vi "Pose3d_getRotation3d.vi"(11 "in Pose3d":T3={"Translation3d"={"X"=0.0, "Y"=0.0, "Z"=0.0}, "Rotation3d"={"Q_quaternion"={"R"=1.0, "V"=[0.0, 0.0, 0.0]}}} {"Translation3d"."Z" format="%14.3f"; "Translation3d"."Y" format="%14.3f"; "Translation3d"."X" format="%14.3f"}) -> (3 "out Rotation3d":T1={"Q_quaternion"={"R"=1.0, "V"=[0.0, 0.0, 0.0]}})   [LabVIEW 2019, in "Trajectory_Library.lvlib"]
doc: "Returns the rotational component of the transformation.\n\nParmeters:\n - IN POSE -- Input POSE data structure\n\nRETURNS:\n - out ROTATION - The rotational component of the pose."
uses:
  Trajectory_Library.lvlib
  POSE3D.ctl
  TRANSLATION3D.ctl
  ROTATION3D.ctl
  QUATERNION.ctl
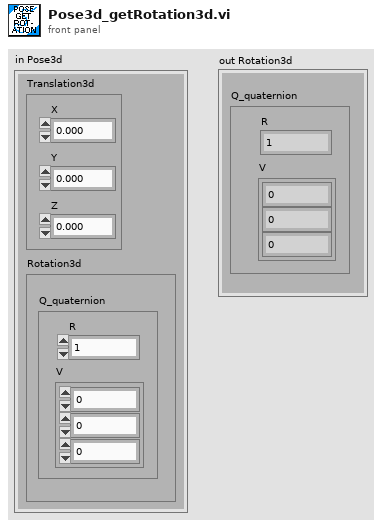
[diagram p1: front panel]
types:
  T1 = typedef "Trajectory_Library.lvlib/ROTATION3D.ctl" = cluster{"Q_quaternion":T2}
  T2 = typedef "Trajectory_Library.lvlib/QUATERNION.ctl" = cluster{"R":dbl, "V":dbl[]}
  T3 = typedef "Trajectory_Library.lvlib/POSE3D.ctl" = cluster{"Translation3d":T4, "Rotation3d":T1}
  T4 = typedef "Trajectory_Library.lvlib/TRANSLATION3D.ctl" = cluster{"X":dbl, "Y":dbl, "Z":dbl}
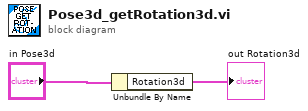
[diagram p0: block diagram]
diagram:
  n1 = Unbundle By Name("in Pose3d") -> ("Rotation3d"=→"out Rotation3d":T1)
